vi "检查更新.vi"(0 "超时ms":dbl) -> (1 "新版本号":string, 2 "新版本号":dbl, 3 "错误?":bool)   [LabVIEW 2017]
uses:
  <vilib>/httpClient/LabVIEWHTTPClient.lvlib
panel:
  out "接收区":string
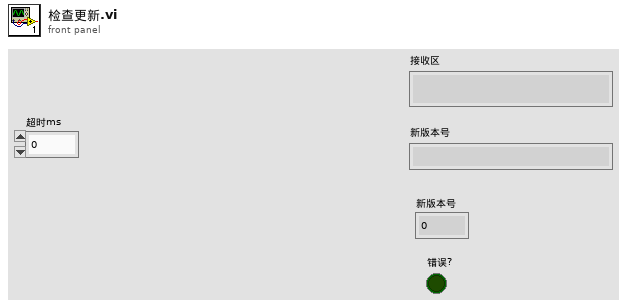
[diagram p1: front panel]
types:
  T1 = typedef "LabVIEWHTTPClient.lvlib/ClientHandle.ctl" = refnum<k1>
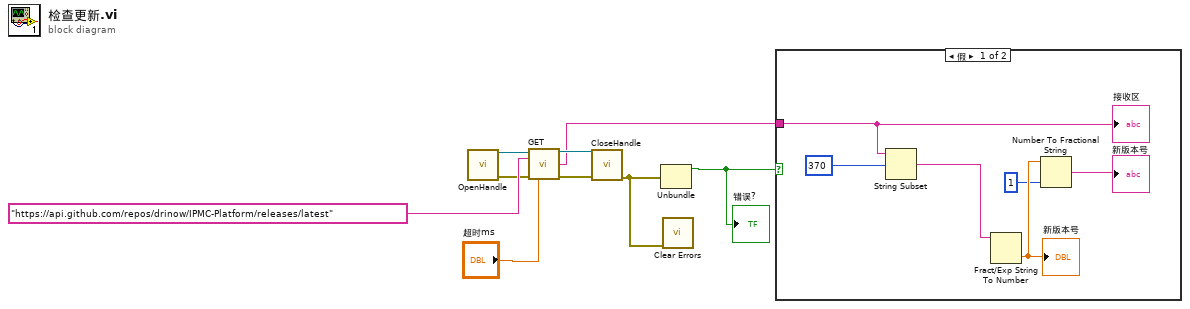
[diagram p0: block diagram]
diagram:
  n1 = call <vilib>:"OpenHandle.vi"() -> ("client handle out"=w9:T1, "error out"=w6:errorcluster)  [unwired: 14 in]
  n2 = call <vilib>:"GET.vi"("client handle"=w9, "url"="https://api.github.com/repos/drinow/IPMC-Platform/releases/latest", "error in (no error)"=w6, "timeout (10000)"="超时ms") -> ("client handle out"=w7:T1, "body"=w4:string, "error out"=w5:errorcluster)  [unwired: 8 in, 1 out]
  n3 = call <vilib>:"CloseHandle.vi"("client handle"=w7, "error in (no error)"=w5) -> ("error out"=w2:errorcluster)  [unwired: 13 in]
  n4 = Unbundle(w2) -> ("status"=w3:bool)  [unwired: 2 out]
  "错误?" <- w3
  n5 = call <vilib>:"Clear Errors.vi"("error in (no error)"=w2) -> ()  [unwired: 5 in, 2 out]
  n6 = case shown="假" w3 {
    tunnel: w4 -> [w15 _]
    frame False {
      n7 = String Subset(string=w15, offset (0)=370) -> (substring=w13:string)  [unwired: 1 in]
      n8 = Fract/Exp String To Number(string=w13) -> (number=w12:dbl)  [unwired: 3 in, 1 out]
      "新版本号" <- w12
      n9 = Number To Fractional String(number=w12, precision (6)=1) -> (F-format string=→"新版本号":string)  [unwired: 2 in]
      "接收区" <- w15
    }
    frame True {
    }
  }
